vi "Pos_Calc Point Move.vi"(8 "Error":errorcluster, 9 "Current Location":T1, 11 "Tartget Location":T1) -> (0 "Error Out":errorcluster, 2 "Down Out":i16, 3 "Right Out":i16)   [LabVIEW 2016]
uses:
  TypeDefs_Utility/Cluster_Pos_Top Left position.ctl
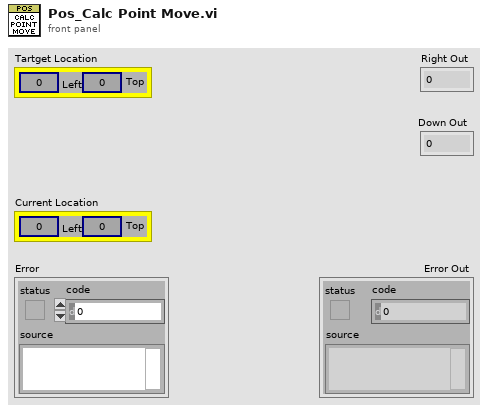
[diagram p1: front panel]
types:
  T1 = typedef "Cluster_Pos_Top Left position.ctl" = cluster{"Left":i16, "Top":i16}
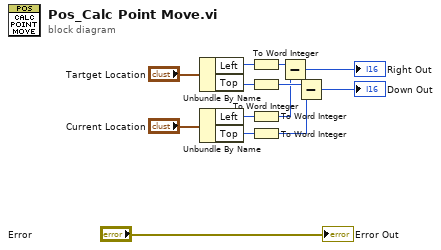
[diagram p0: block diagram]
diagram:
  n1 = Unbundle By Name("Tartget Location") -> ("Left"=w11:i16, "Top"=w8:i16)
  n2 = Unbundle By Name("Current Location") -> ("Left"=w10:i16, "Top"=w7:i16)
  n3 = To Word Integer(number=w11) -> (16bit integer=w5:i16)
  n4 = To Word Integer(number=w8) -> (16bit integer=w4:i16)
  n5 = To Word Integer(number=w10) -> (16bit integer=w3:i16)
  n6 = To Word Integer(number=w7) -> (16bit integer=w2:i16)
  n7 = Subtract(x=w5, y=w3) -> (x-y=→"Right Out":i16)
  n8 = Subtract(x=w4, y=w2) -> (x-y=→"Down Out":i16)
  "Error Out" <- "Error"
